vi "IndexSettingsCluster.vi"(11 "Names Array":string[][](array[string])) -> (3 "index Array":i32[][](array[numeric]))   [LabVIEW 2011]
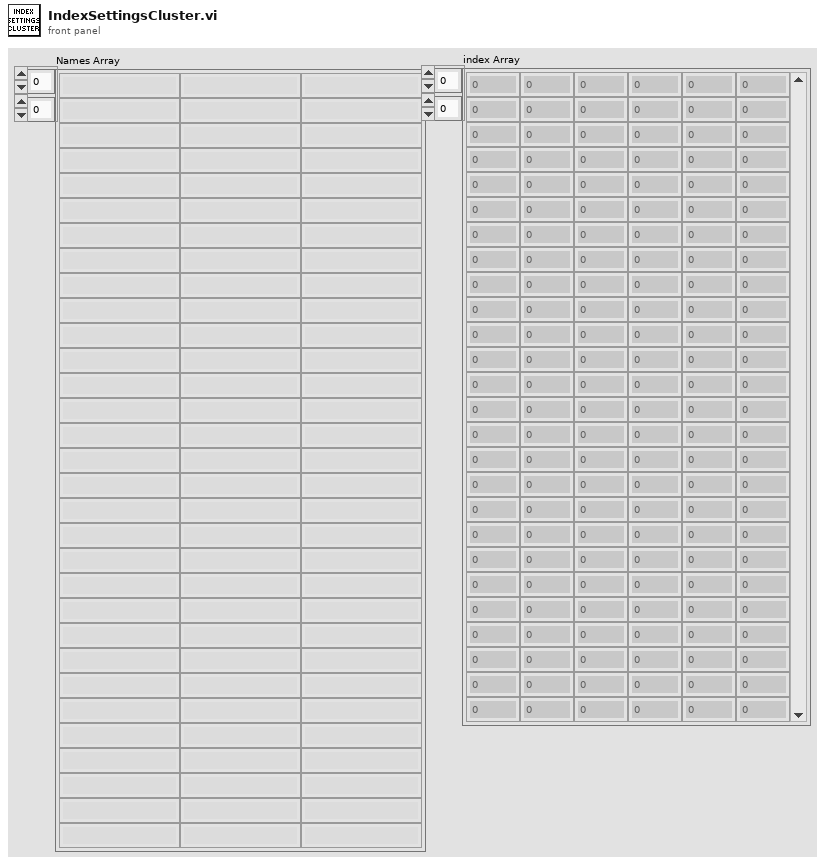
[diagram p1: front panel]
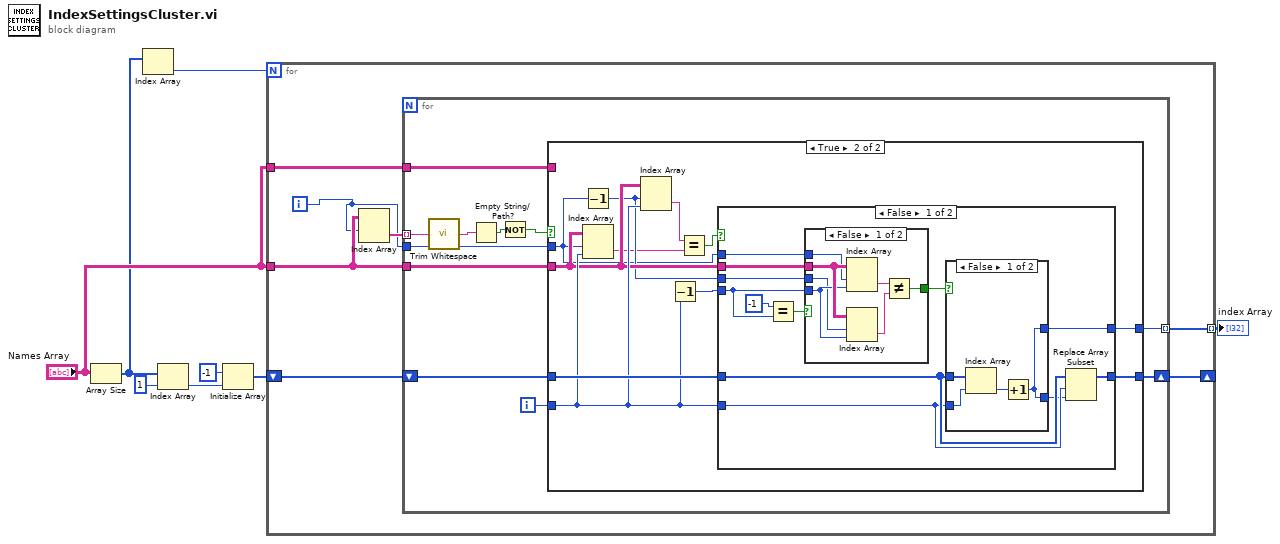
[diagram p0: block diagram]
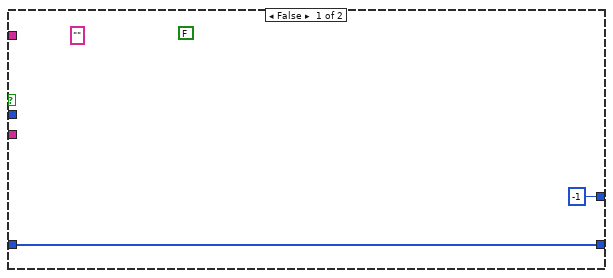
[diagram p2: hidden frame]
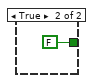
[diagram p3: hidden frame]
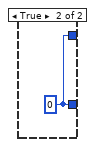
[diagram p4: hidden frame]
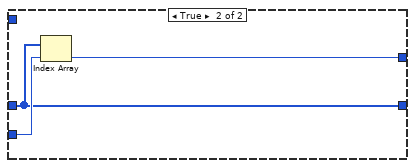
[diagram p5: hidden frame]
diagram:
  n1 = Array Size(array="Names Array") -> (size(s)=w3:i32[])
  n2 = Index Array(array=w3) -> (element=w1:i32)  [unwired: 1 in]
  n3 = Index Array(array=w3, index=1) -> (element=w2:i32)
  n4 = Initialize Array(-1, w2) -> (w6:i32[])
  n5 = for {
    N: w1 -> [_]
    shift-right: [w13] -> _
    shift-left: w6 -> [w15]
    tunnel: "Names Array" -> [w14]
    tunnel: [w11] -> w5 mode=indexing
    tunnel: "Names Array" -> [w10]
    i -> [w9]
    n6 = Index Array(array=w10, index (row)=w9) -> (element=w12:string[])  [unwired: 1 in]
    n7 = for {
      tunnel: w12 -> [w17] mode=indexing
      shift-right: [w23] -> w13
      shift-left: w15 -> [w24]
      tunnel: w14 -> [w25]
      tunnel: w9 -> [w26]
      tunnel: [w20] -> w11 mode=indexing
      tunnel: w10 -> [w19]
      i -> [w18]
      n8 = call "Trim Whitespace.vi"("string"=w17) -> ("trimmed string"=w16:string)  [unwired: 1 in]
      n9 = Empty String/Path?(string/path=w16) -> (empty?=w22:bool)
      n10 = Not(x=w22) -> (.not. x?=w21:bool)
      n11 = case shown="True" w21 {
        tunnel: w26 -> [_ w32]
        tunnel: w25 -> [_ _]
        tunnel: w24 -> [w27 w39]
        tunnel: [w27 w38] -> w23
        tunnel: [-1 ("t") w37] -> w20
        tunnel: w19 -> [_ w35]
        tunnel: w18 -> [_ w36]
        frame False {
          (unwired) FALSE
          (unwired) ""
        }
        frame True {
          n12 = Decrement(x=w32) -> (x-1=w33:i32)
          n13 = Index Array(array=w35, index (row)=w32, index (col)=w36) -> (element=w30:string)
          n14 = Index Array(array=w35, index (row)=w33, index (col)=w36) -> (element=w31:string)
          n15 = Decrement(x=w36) -> (x-1=w34:i32)
          n16 = Equal?(x=w31, y=w30) -> (x = y?=w29:bool)
          n17 = case shown="False" w29 {
            tunnel: w39 -> [w50 w65]
            tunnel: w36 -> [w49 w67]
            tunnel: [w51 w65] -> w38
            tunnel: [w47 w66] -> w37
            tunnel: w35 -> [w46 _]
            tunnel: w34 -> [w42 _]
            tunnel: w33 -> [w45 _]
            tunnel: w32 -> [w44 _]
            frame False {
              n18 = Equal?(x=-1, y=w42) -> (x = y?=w40:bool)
              n19 = case shown="False" w40 {
                tunnel: w46 -> [w58 _]
                tunnel: w42 -> [w57 _]
                tunnel: w45 -> [w56 _]
                tunnel: w44 -> [w55 _]
                tunnel: [w52 FALSE] -> w43
                frame False {
                  n20 = Index Array(array=w58, index (row)=w55, index (col)=w57) -> (element=w54:string)
                  n21 = Index Array(array=w58, index (row)=w56, index (col)=w57) -> (element=w53:string)
                  n22 = Not Equal?(x=w54, y=w53) -> (x != y?=w52:bool)
                }
                frame True {
                }
              }
              n23 = case shown="False" w43 {
                tunnel: w50 -> [w63 _]
                tunnel: w49 -> [w62 _]
                tunnel: [w60 w64] -> w48
                tunnel: [w60 w64] -> w47
                frame False {
                  n24 = Index Array(array=w63, index=w62) -> (element=w61:i32)
                  n25 = Increment(x=w61) -> (x+1=w60:i32)
                }
                frame True {
                  w64 = 0
                }
              }
              n26 = Replace Array Subset(array=w50, new element=w48, index=w49) -> (w51:i32[])
            }
            frame True {
              n27 = Index Array(array=w65, index=w67) -> (element=w66:i32)
            }
          }
        }
      }
    }
  }
  "index Array" <- w5
